vi "Find_Old_ID&ChangeTo_Min-1.vi"(1 "track ID OLD":u16, 2 "track ID (min)":u16, 3 "ID-dot col IN":u16[](array[numeric])) -> (0 "ID-dot col OUT":u16[](array[numeric]))   [LabVIEW 2013]
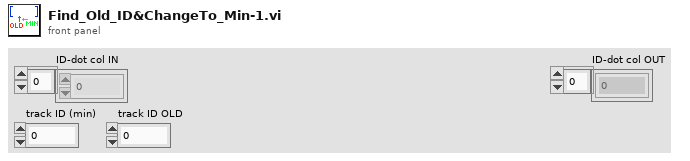
[diagram p1: front panel]
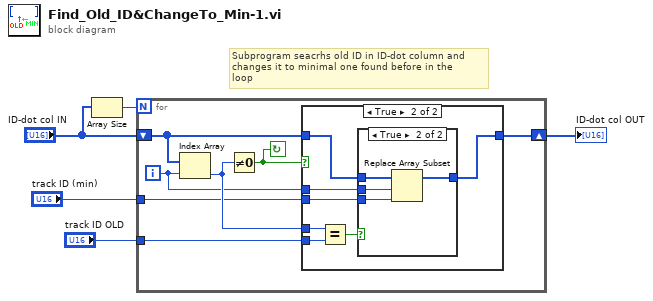
[diagram p0: block diagram]
diagram:
  # "Subprogram seacrhs old ID in ID-dot column and \nchanges it to minimal one found before in the \nloop"
  n1 = Array Size(array="ID-dot col IN") -> (size(s)=w5:i32)
  n2 = for {
    N: w5 -> [_]
    shift-right: [w6] -> w1
    shift-left: "ID-dot col IN" -> [w11]
    tunnel: "track ID OLD" -> [w10]
    tunnel: "track ID (min)" -> [w7]
    i -> [w8]
    stop <- w12 continue-if-true
    n3 = Index Array(array=w11, index=w8) -> (element=w9:u16)
    n4 = Not Equal To 0?(x=w9) -> (x != 0?=w12:bool)
    n5 = case shown="True" w12 {
      tunnel: w11 -> [w13 w17]
      tunnel: w10 -> [_ w19]
      tunnel: w9 -> [_ w20]
      tunnel: w8 -> [_ w16]
      tunnel: w7 -> [_ w15]
      tunnel: [w13 w14] -> w6
      frame False {
      }
      frame True {
        n6 = Equal?(x=w20, y=w19) -> (x = y?=w18:bool)
        n7 = case shown="True" w18 {
          tunnel: w17 -> [w21 w25]
          tunnel: w16 -> [_ w24]
          tunnel: w15 -> [_ w23]
          tunnel: [w21 w22] -> w14
          frame False {
          }
          frame True {
            n8 = Replace Array Subset(array=w25, new element=w23, index=w24) -> (w22:u16[])
          }
        }
      }
    }
  }
  "ID-dot col OUT" <- w1
